vi "Write Row of Data to Excel Spreadsheet 2010.vi"() -> ()   [LabVIEW 2015]
uses:
  <vilib>/Utility/file.llb/Write Delimited Spreadsheet (DBL).vi
  <vilib>/Utility/NIReport.llb/Append Numeric Table to Report (wrap).vi
  <vilib>/Utility/NIReport.llb/NI_report.lvclass
  <vilib>/Utility/NIReport.llb/Excel/NI_Excel.lvclass
panel:
  in  "stop":bool
  in  "Excel File":path
  # "Select an Excel file to append new data to. Run this VI \nmultiple times to append multiple rows of random data \nto a spreadsheet."
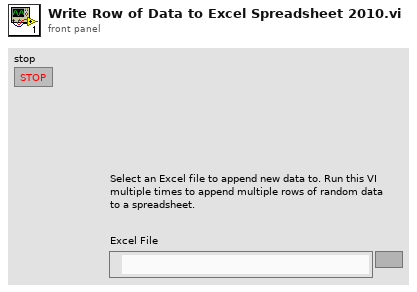
[diagram p1: front panel]
types:
  T1 = enum16{"Standard Report", "HTML", "Word", "Excel"}
  T2 = cluster{"position (Excel)":cluster{"row":i32, "column":i32}, "name (Excel)":string, "bookmark (Word)":string}
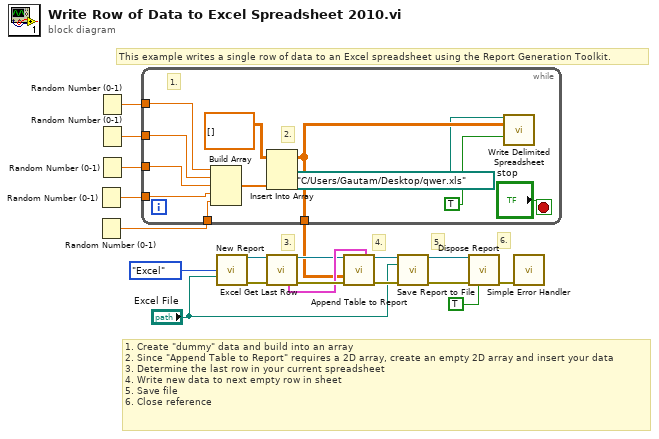
[diagram p0: block diagram]
diagram:
  # "This example writes a single row of data to an Excel spreadsheet using the Report Generation Toolkit."
  # "1. Create \"dummy\" data and build into an array\n2. Since \"Append Table to Report\" requires a 2D array, create an empty 2D array and insert your data\n3. Determine the last row in your current spreadsheet \n4. Write new data to next empty row in sheet\n5. Save file\n6. Close reference"
  # "6."
  # "5."
  # "4."
  # "3."
  n1 = Random Number (0-1)() -> (number: 0 to 1=w3:dbl)
  n2 = Random Number (0-1)() -> (number: 0 to 1=w2:dbl)
  n3 = Random Number (0-1)() -> (number: 0 to 1=w6:dbl)
  n4 = Random Number (0-1)() -> (number: 0 to 1=w5:dbl)
  n5 = Random Number (0-1)() -> (number: 0 to 1=w4:dbl)
  n6 = while {
    tunnel: w6 -> [w29]
    tunnel: w5 -> [w28]
    tunnel: w4 -> [w27]
    tunnel: w3 -> [w26]
    tunnel: w2 -> [w25]
    tunnel: [w23] -> w1
    stop <- "stop" stop-if-true
    # "2."
    # "1."
    n7 = Build Array(w29, w28, w27, w26, w25) -> (w24:dbl[])
    n8 = Insert Into Array(array=dbl[][] [], new element=w24) -> (w23:dbl[][])  [unwired: 2 in]
    n9 = call-poly <vilib>:"Write Delimited Spreadsheet.vi"("file path (dialog if empty)"=path "C:/Users/Gautam/Desktop/qwer.xls", "2D data"=w23, "append to file? (F)"=TRUE) -> ()  [unwired: 11 in, 2 out]
  }
  n10 = call <vilib>:"New Report.vi"("report type"=T1."Excel", "template (empty)"="Excel File") -> ("report out"=w19:refnum<class "NI_report.lvclass">, "error out"=w17:errorcluster)  [unwired: 12 in]
  n11 = call <vilib>:"Excel Get Last Row.vi"("report in"=w19, "error in (no error)"=w17) -> ("report out"=w8:refnum<class "NI_report.lvclass">, "MS Office parameters out"=w15:T2, "error out"=w16:errorcluster)  [unwired: 11 in]
  n12 = call-poly <vilib>:"Append Table to Report.vi"("report in"=w8, "MS Office parameters"=w15, "numerical data"=w1, "error in (no error)"=w16) -> ("report out"=w10:refnum<class "NI_report.lvclass">, "error out"=w9:errorcluster)  [unwired: 8 in, 2 out]
  n13 = call-dynamic "Save Report to File.vi"("report in"=w10, "report file path"="Excel File", "error in (no error)"=w9) -> ("report out"=w12:refnum<class "NI_report.lvclass">, "error out"=w11:errorcluster)  [unwired: 11 in]
  n14 = call-dynamic "Dispose Report.vi"("report in"=w12, "error in (no error)"=w11, "close report? (T)"=TRUE ("Close Report? (T)")) -> ("error out"=w14:errorcluster)  [unwired: 2 in, 10 out]
  n15 = call <vilib>:"Simple Error Handler.vi"("error in (no error)"=w14) -> ()  [unwired: 1 in, 8 out]
